vi "test_libssh2_session_blocking.vi"() -> ()   [LabVIEW 2013, in "libssh2_integration_tests.lvlib"]
uses:
  libssh2_integration_tests.lvlib
  <vilib>/addons/_JKI Toolkits/Caraya/classes/Test/Test.lvclass
  libssh2/libssh2.lvlib
  <vilib>/addons/_JKI Toolkits/Caraya/classes/Assert/Assert.lvclass
panel:
  out "error out":errorcluster
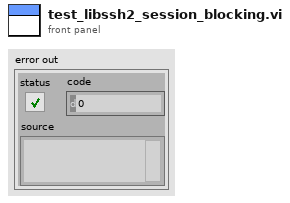
[diagram p1: front panel]
types:
  T1 = typedef "libssh2.lvlib/Session Refnum.ctl" = refnum<k1>
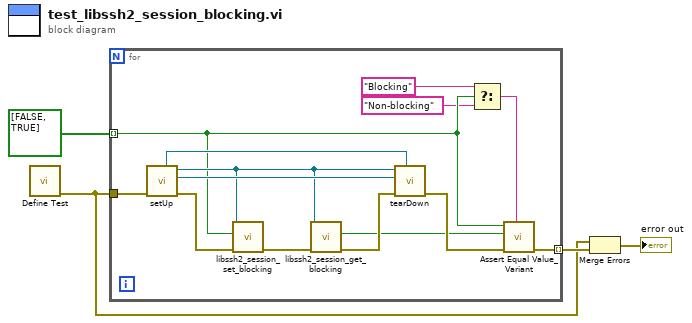
[diagram p0: block diagram]
diagram:
  n1 = call <vilib>:"Define Test.vi"() -> ("error out"=w2:errorcluster)  [unwired: 10 in, 1 out]
  n2 = for {
    tunnel: [w18] -> w4 mode=indexing
    tunnel: w2 -> [w17]
    tunnel: bool[] [FALSE, TRUE] -> [w8] mode=indexing
    n3 = call "setUp.vi"("error in (no error)"=w17) -> ("error out"=w13:errorcluster, "connection ID"=w16:refnum<k5>, "session"=w10:T1, "fixture"=w15:refnum<class "Server Fixture.lvclass">)  [unwired: 7 in]
    n4 = call "libssh2_session_set_blocking.vi"("error in (no error)"=w13, "blocking"=w8, "session"=w10) -> ("error out"=w14:errorcluster)  [unwired: 8 in]
    n5 = call "libssh2_session_get_blocking.vi"("error in (no error)"=w14, "session"=w10) -> ("error out"=w11:errorcluster, "blocking"=w9:bool)  [unwired: 8 in]
    n6 = call "tearDown.vi"("fixture"=w15, "error in (no error)"=w11, "connection ID"=w16, "session"=w10) -> ("error out"=w12:errorcluster)  [unwired: 7 in]
    n7 = Select(t="Blocking", s=w8, f="Non-blocking") -> (s? t:f=w5:string)
    n8 = call <vilib>:"Assert Equal Value_Variant.vi"("Label"=w5, "error in (no error)"=w12, "Y"=w9, "X"=w8) -> ("error out"=w18:errorcluster)  [unwired: 6 in, 1 out]
  }
  n9 = Merge Errors(w2, w4) -> (→"error out":errorcluster)
